vi "Reinitialize Sample Period Control.vi"(4 "error in (no error)":errorcluster, 6 "Plugin Names":T1, 7 "Digital in":refnum<vi>) -> (0 "error out":errorcluster)   [LabVIEW 2015, in "Startup Processes.lvlib"]
uses:
  Startup Processes.lvlib
  _typedefs/Subpanel Names.ctl
  _buffers/Sample Rate/Sample Rate.lvlib
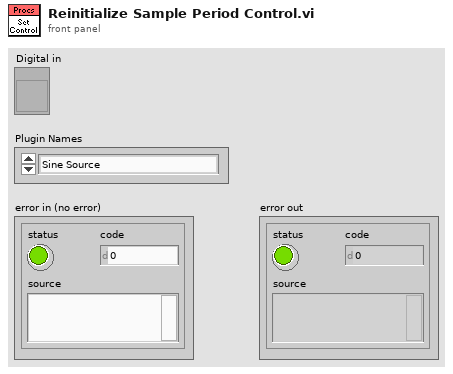
[diagram p1: front panel]
types:
  T1 = typedef "Startup Processes.lvlib/Subpanel Names.ctl" = enum16{"Sine Source", "Ramp Source", "Hen House TC", "Dog House TC", "Out House TC"}
  T2 = enum8{"Enabled", "Disabled", "Disabled and Grayed Out"}
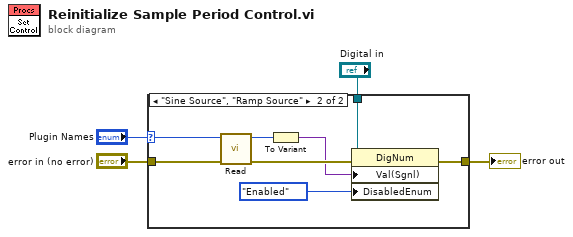
[diagram p0: block diagram]
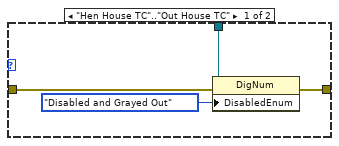
[diagram p2: hidden frame]
diagram:
  n1 = case shown="\"Sine Source\", \"Ramp Source\"" "Plugin Names" {
    selector: "Plugin Names" -> [_ w13]
    tunnel: "Digital in" -> [w8 w16]
    tunnel: "error in (no error)" -> [w7 w12]
    tunnel: [w6 w15] -> w1
    frame "Hen House TC".."Out House TC" {
      n2 = property on="Property Node" class="DigNum"(reference=w8, error in=w7, "DisabledEnum"=T2."Disabled and Grayed Out" ("Disabled")) -> (error out=w6:errorcluster)  [unwired: 1 out]
    }
    frame "Sine Source", "Ramp Source" {
      n3 = call "Read.vi"("Error In"=w12, "Plugin Name"=w13) -> ("Error Out"=w11:errorcluster, "Sample Period (msec)"=w10:i32)  [unwired: 4 in]
      n4 = To Variant(anything=w10) -> (Variant=w9:variant)
      n5 = property on="Property Node" class="DigNum"(reference=w16, error in=w11, "Val(Sgnl)"=w9, "DisabledEnum"=T2."Enabled" ("Disabled")) -> (error out=w15:errorcluster)  [unwired: 1 out]
    }
  }
  "error out" <- w1
